vi "Error to String 2012 NIVerified.vi"(10 "Error Array":errorcluster[](array[cluster]), 11 "Error In":errorcluster) -> (2 "Errors Strings":string, 3 "Errors status":bool)   [LabVIEW 2024]
doc: "Converts error message(s) to a string. Can accept a single error message, an array of error messages, or both. Unlike the 'Merge Errors.vi', this VI actually combines ALL of the errors that occured into one long string.\n\nError in - Single error message cluster in\nError Array - Array of error message clusters in\n\nStatus - Indicates error status. True indicates error has occured.\nError String - A string of all the error codes, conditions, and messages concatenated into one long string."
uses:
  <vilib>/Utility/error.llb/DialogType.ctl
panel:
  # "Overview: This example converts a single error to a string or an array of errors while only writing errors that have occurred\nRequirements: LabVIEW Full Development System 2012 or compatible\nInstructions:\n1- Modifying the Status and Code on the Error In or Error Array Clusters\n2- Run the VI\n3- Notice that the  errors are concatenated in the Errors Strings and the Error status turns ON if any error occurs"
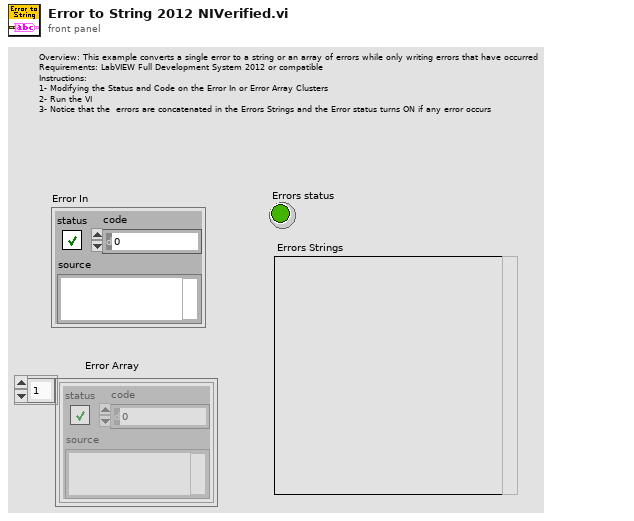
[diagram p1: front panel]
types:
  T1 = typedef "DialogType.ctl" = u16
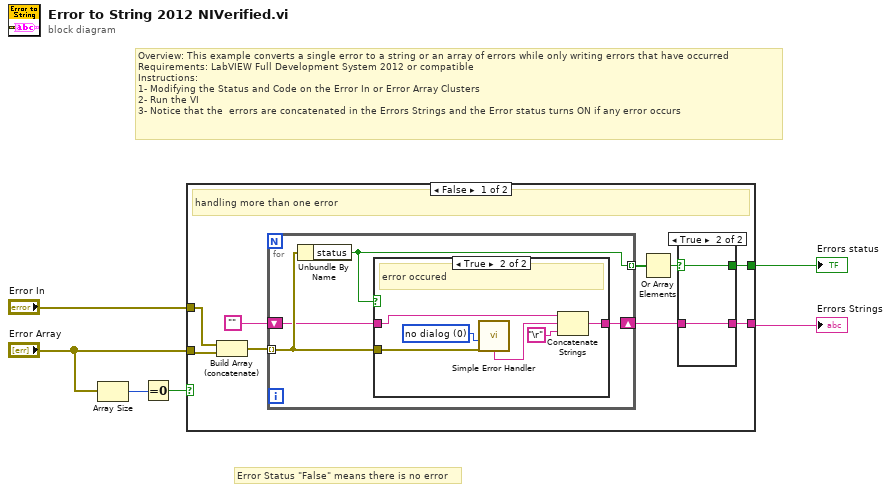
[diagram p0: block diagram]
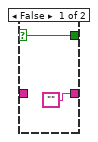
[diagram p2: hidden frame]
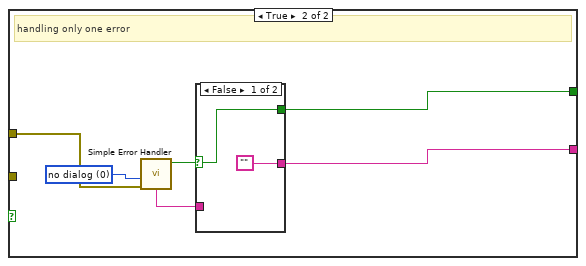
[diagram p4: hidden frame]
diagram:
  # "Overview: This example converts a single error to a string or an array of errors while only writing errors that have occurred\nRequirements: LabVIEW Full Development System 2012 or compatible\nInstructions:\n1- Modifying the Status and Code on the Error In or Error Array Clusters\n2- Run the VI\n3- Notice that the  errors are concatenated in the Errors Strings and the Error status turns ON if any error occurs"
  # "Error Status \"False\" means there is no error"
  n1 = Array Size(array="Error Array") -> (size(s)=w3:i32)
  n2 = Equal To 0?(x=w3) -> (x = 0?=w2:bool)
  n3 = case shown="False" w2 {
    tunnel: "Error In" -> [w7 w35]
    tunnel: [w9 w33] -> w5
    tunnel: [w11 w34] -> w4
    tunnel: "Error Array" -> [w13 _]
    frame False {
      # "handling more than one error"
      n4 = Build Array (concatenate)(w7, w13) -> (w15:errorcluster[])
      n5 = for {
        tunnel: w15 -> [w23] mode=indexing
        shift-right: [w22] -> w10
        shift-left: "" -> [w21]
        tunnel: [w20] -> w14 mode=indexing
        n6 = Unbundle By Name(w23) -> ("status"=w20:bool)
        n7 = case shown="True" w20 {
          tunnel: w23 -> [_ w30]
          tunnel: [w24 w28] -> w22
          tunnel: w21 -> [w24 w29]
          frame False {
            # "no error occured"
          }
          frame True {
            w25 = T1 0 items=["no dialog", "OK message", "continue or stop message", "OK message + warnings", "continue/stop + warnings"] ("type of dialog (OK msg:1)")
            # "error occured"
            n8 = call <vilib>:"Simple Error Handler.vi"("type of dialog (OK msg:1)"=w25, "error in (no error)"=w30) -> ("message"=w27:string)  [unwired: 3 in, 4 out]
            n9 = Concatenate Strings(w29, w27, "\r") -> (w28:string)
          }
        }
      }
      n10 = Or Array Elements(Boolean array=w14) -> (logical OR=w12:bool)
      n11 = case shown="True" w12 {
        selector: w12 -> [w17 w18]
        tunnel: ["" w19] -> w11
        tunnel: w10 -> [_ w19]
        tunnel: [w17 w18] -> w9
        frame False {
        }
        frame True {
        }
      }
    }
    frame True {
      w36 = T1 0 items=["no dialog", "OK message", "continue or stop message", "OK message + warnings", "continue/stop + warnings"] ("type of dialog (OK msg:1)")
      # "handling only one error"
      n12 = call <vilib>:"Simple Error Handler.vi"("type of dialog (OK msg:1)"=w36, "error in (no error)"=w35) -> ("error?"=w31:bool, "message"=w32:string)  [unwired: 3 in, 3 out]
      n13 = case shown="False" w31 {
        selector: w31 -> [w38 w39]
        tunnel: ["" w40] -> w34
        tunnel: w32 -> [_ w40]
        tunnel: [w38 w39] -> w33
        frame False {
        }
        frame True {
        }
      }
    }
  }
  "Errors status" <- w5
  "Errors Strings" <- w4
